vi "Module - Calibration.vi"(8 "Error In":errorcluster) -> (0 "Error Out":errorcluster)   [LabVIEW 2020]
uses:
  Control/State - Calibration.ctl
  Control/Cluster - Calibration Data.ctl
  Control/State - eFGV.ctl
  Control/Section Config RT.ctl
  <vilib>/Analysis/baseanly.llb/Mean (DBL).vi
  <vilib>/Analysis/NI_AALBase.lvlib
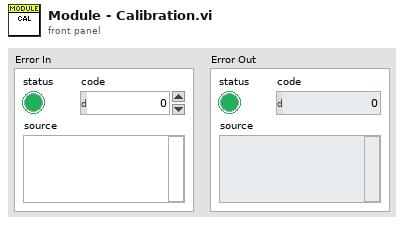
[diagram p1: front panel]
types:
  T1 = typedef "Cluster - Calibration Data.ctl" = cluster{"Slope":sgl, "Intercept":sgl, "Offset":sgl}
  T2 = cluster{"T_Out":i32, "AI Agg":waveform(dbl)[], "Calibration Data":T1[], "AI Calibrated":sgl[], "Event Ref":refnum<event-registration>, "Event - NS Connected":bool}
  T3 = typedef "State - Calibration.ctl" = enum16{"Init", "Register Event", "Read Calibration Config", "Idle", "Calibrate Sensor", "Close"}
  T4 = typedef "State - eFGV.ctl" = enum16{"Init", "Read", "Write", "Exit"}
  T5 = typedef "Section Config RT.ctl" = enum16{"Mod1/AI0", "Mod1/AI1", "Mod1/AI2", "Mod1/AI3", "Network Stream", "Acquisition Setting"}
  T6 = enum32{"invalid app kind", "Development System", "Run Time System", "Student Edition", "Embedded LabVIEW", "Evaluation", "Custom"}
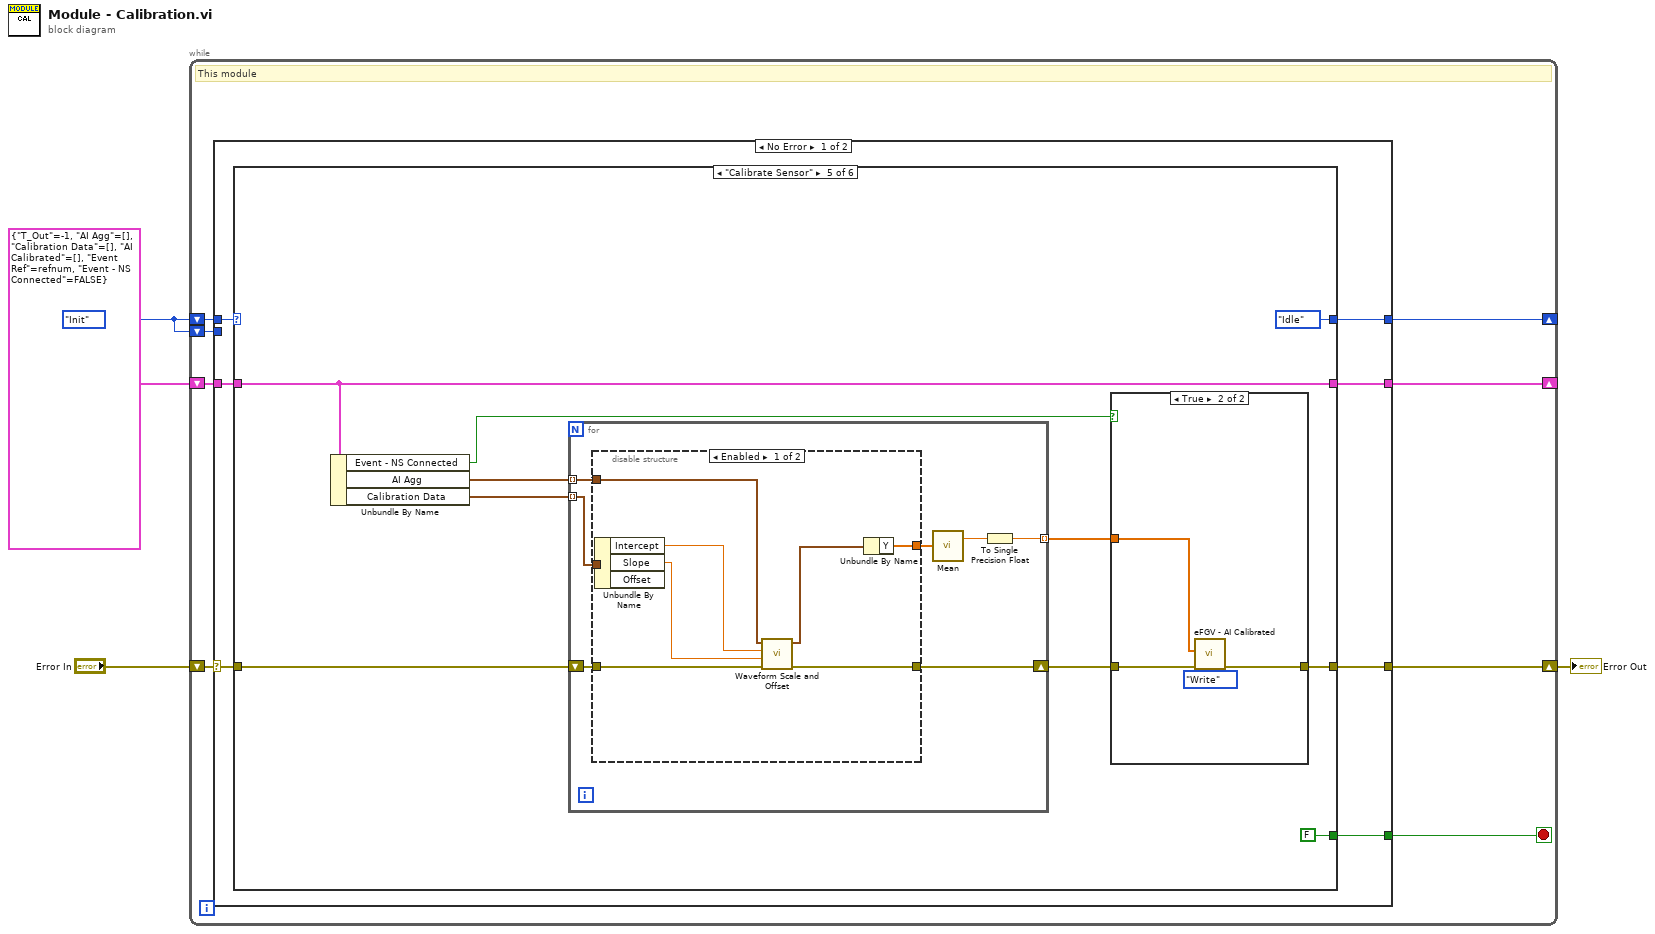
[diagram p0: block diagram]
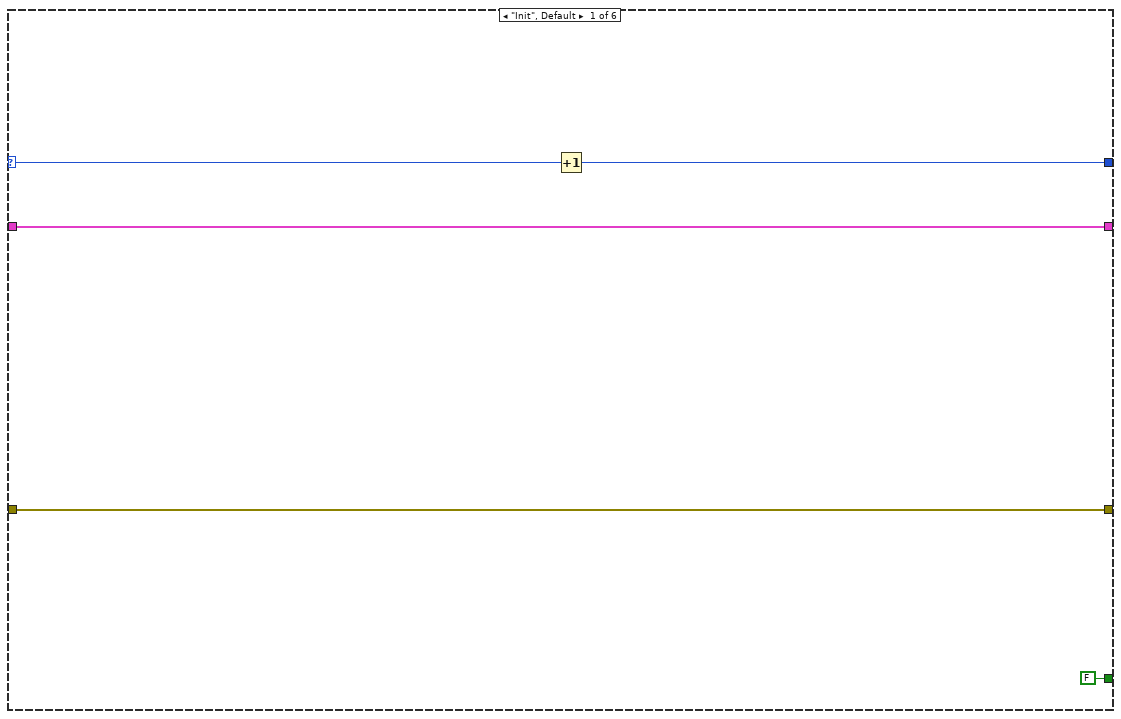
[diagram p2: hidden frame]
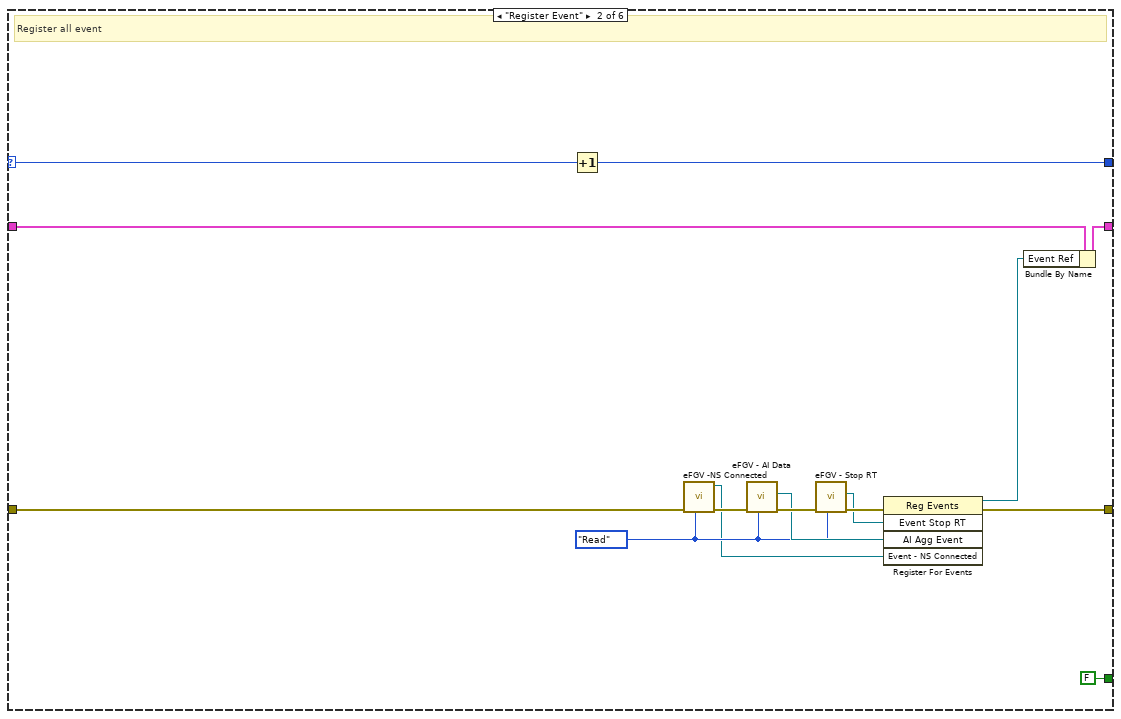
[diagram p3: hidden frame]
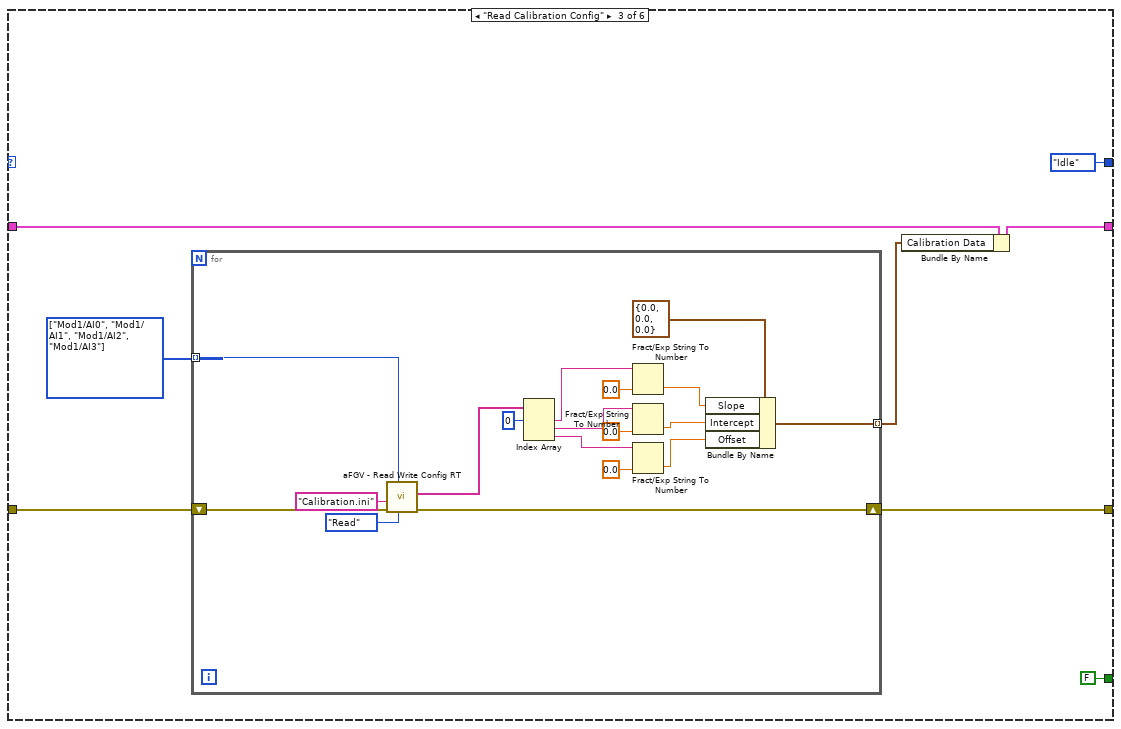
[diagram p4: hidden frame]
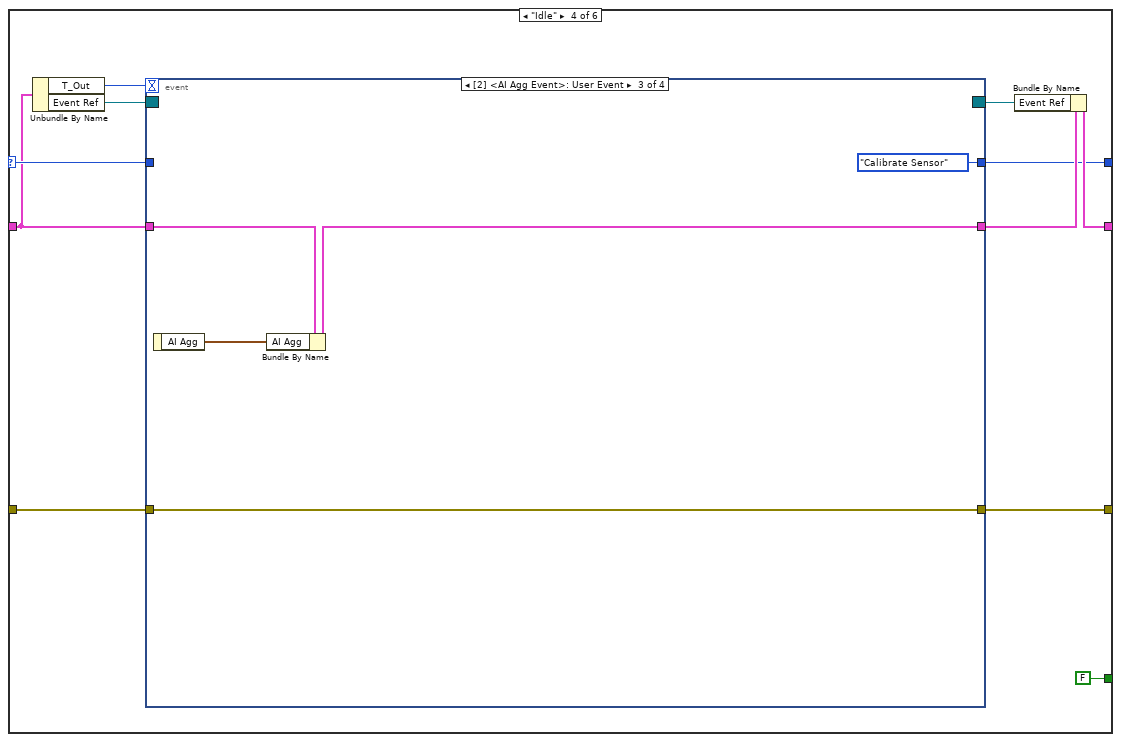
[diagram p5: hidden frame]
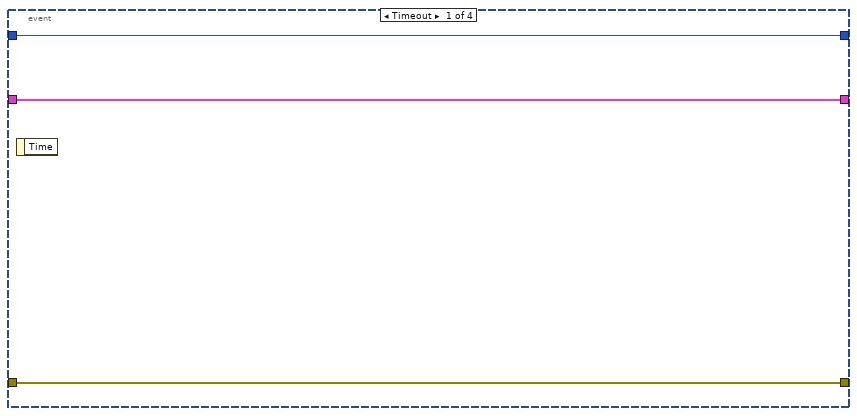
[diagram p6: hidden frame]
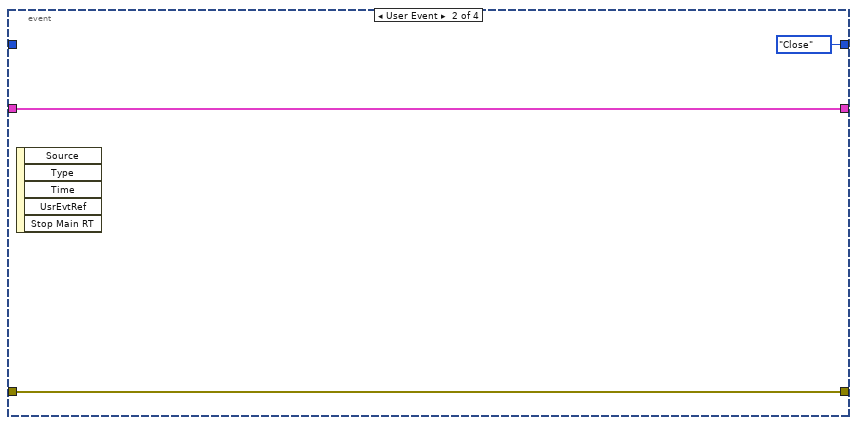
[diagram p7: hidden frame]
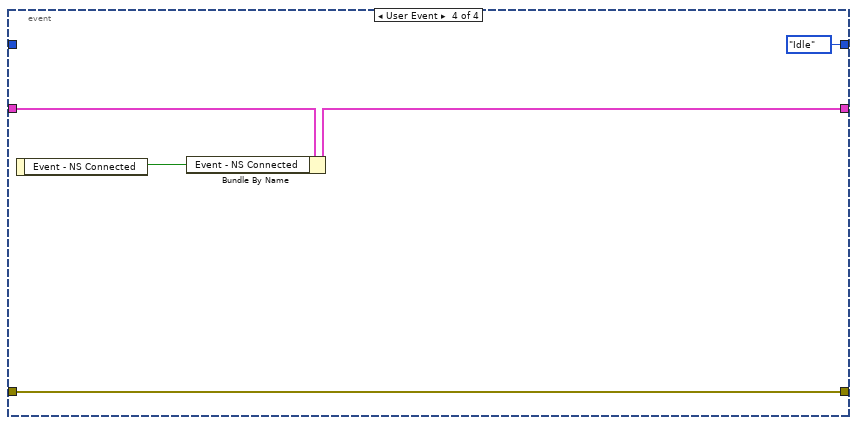
[diagram p8: hidden frame]
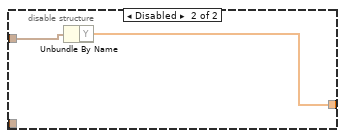
[diagram p10: hidden frame]
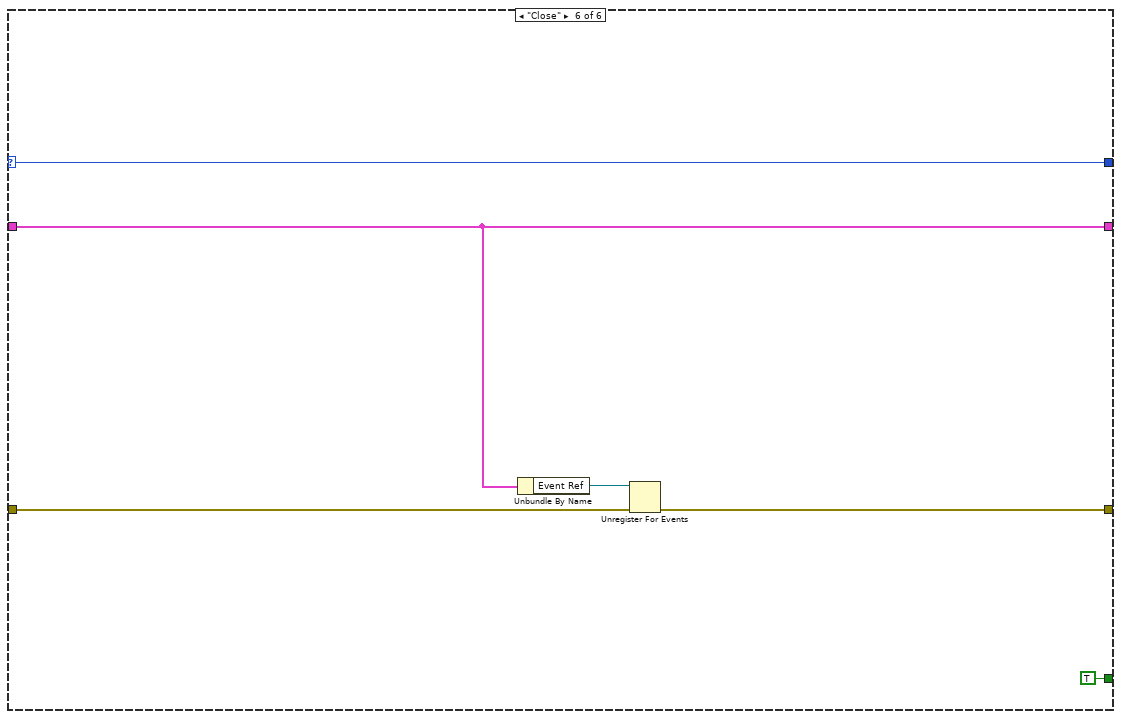
[diagram p11: hidden frame]
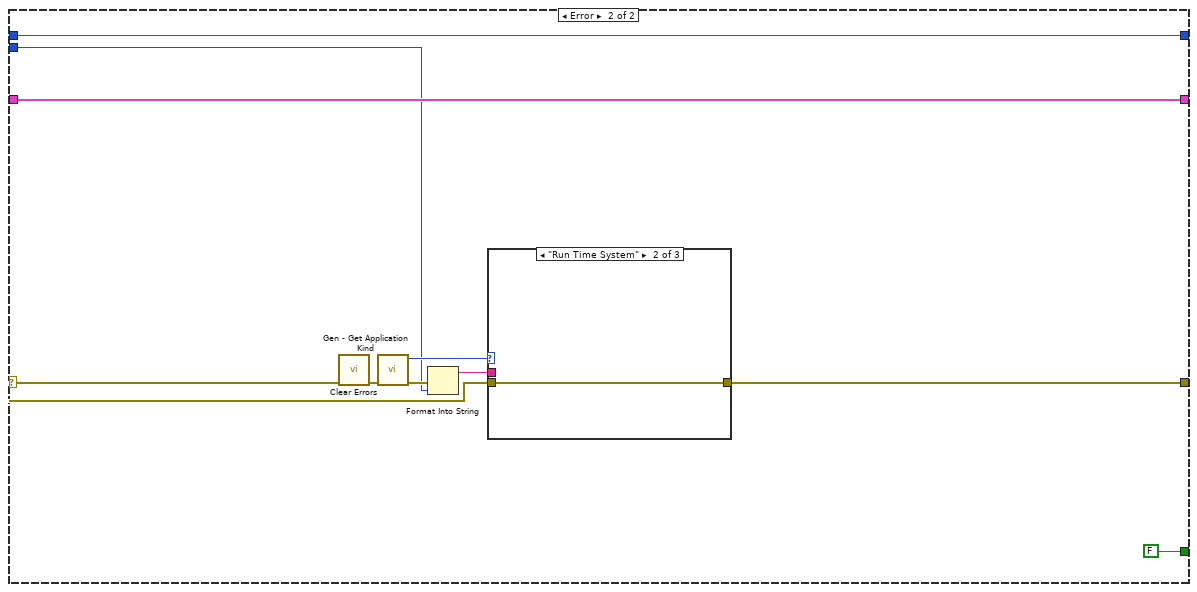
[diagram p12: hidden frame]
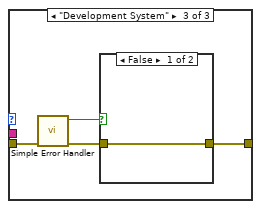
[diagram p14: hidden frame]
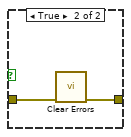
[diagram p15: hidden frame]
diagram:
  w1 = State_-_Calibration."Init"
  n1 = while {
    shift-right: [w8] -> _
    shift-left: w1 -> [w10]
    shift-right: [w11] -> w3
    shift-left: "Error In" -> [w12]
    shift-right: [w6] -> _
    shift-left: T2 {"T_Out"=-1, "AI Agg"=[], "Calibration Data"=[], "AI Calibrated"=[], "Event Ref"=refnum, "Event - NS Connected"=FALSE} -> [w7]
    shift-left: w1 -> [w5]
    stop <- w9 stop-if-true
    # "This module"
    n2 = case shown="No Error" w12 {
      selector: w12 -> [w19 w138]
      tunnel: w10 -> [w18 w135]
      tunnel: [w14 w139] -> w11
      tunnel: [w17 FALSE] -> w9
      tunnel: [w13 w135] -> w8
      tunnel: w7 -> [w16 w134]
      tunnel: [w15 w134] -> w6
      tunnel: w5 -> [_ w132]
      frame No Error {
        n3 = case shown="\"Calibrate Sensor\"" w18 {
          selector: w18 -> [w21 w31 _ w72 _ w128]
          tunnel: [w24 w39 w43 w76 w95 w129] -> w14
          tunnel: w19 -> [w24 w28 w44 w75 w99 w130]
          tunnel: [FALSE FALSE FALSE FALSE FALSE TRUE] -> w17
          tunnel: [w20 w30 State_-_Calibration."Idle" w66 State_-_Calibration."Idle" w128] -> w13
          tunnel: w16 -> [w23 w35 w47 w71 w100 w126]
          tunnel: [w23 w34 w41 w68 w100 w126] -> w15
          frame "Init", Default {
            n4 = Increment(x=w21) -> (x+1=w20:T3)
          }
          frame "Register Event" {
            w27 = State_-_eFGV."Read" ("State")
            # "Register all event"
            n5 = Increment(x=w31) -> (x+1=w30:T3)
            n6 = call "eFGV -NS Connected.vi"("States"=w27, "Error In"=w28) -> ("Error Out"=w29:errorcluster, "Event - NS Connected"=w26:refnum<user-event>)  [unwired: 8 in]
            n7 = call "eFGV - AI Data.vi"("States"=w27, "Error In"=w29) -> ("Error Out"=w33:errorcluster, "AI Agg Event"=w32:refnum<user-event>)  [unwired: 8 in]
            n8 = call "eFGV - Stop RT.vi"("State"=w27, "Error In"=w33) -> ("Error Out"=w38:errorcluster, "Event Stop RT"=w36:refnum<user-event>)  [unwired: 7 in, 1 out]
            n9 = register-events(error in=w38, w36, w32, w26) -> (reference out=w25:refnum<event-registration>, error out=w39:errorcluster)  [unwired: 1 in]
            n10 = Bundle By Name(cluster=w35, "Event Ref"=w25) -> (w34:T2)
          }
          frame "Read Calibration Config" {
            w42 = T5[] [enum."Mod1/AI0", enum."Mod1/AI1", enum."Mod1/AI2", enum."Mod1/AI3"] items=["Mod1/AI0", "Mod1/AI1", "Mod1/AI2", "Mod1/AI3", "Network Stream", "Acquisition Setting"] ("Array")
            n11 = for {
              shift-right: [w64] -> w43
              shift-left: w44 -> [w65]
              tunnel: w42 -> [w52] mode=indexing
              tunnel: [w48] -> w40 mode=indexing
              n12 = call "aFGV - Read Write Config RT.vi"("State"=enum16{"Read", "Write", "Delete"}."Read", "Section"=w52, "Error In"=w65, "File name"="Calibration.ini") -> ("Error Out"=w64:errorcluster, "Data out"=w62:string[])  [unwired: 5 in, 1 out]
              n13 = Index Array(array=w62, index #1=0 ("index")) -> (element #1=w51:string, element #2=w50:string, element #3=w49:string)  [unwired: 2 in]
              n14 = Fract/Exp String To Number(string=w51, default (0 dbl)=sgl 0.0 ("default (0 DBL)")) -> (number=w56:sgl)  [unwired: 2 in, 1 out]
              n15 = Fract/Exp String To Number(string=w50, default (0 dbl)=sgl 0.0 ("default (0 DBL)")) -> (number=w55:sgl)  [unwired: 2 in, 1 out]
              n16 = Fract/Exp String To Number(string=w49, default (0 dbl)=sgl 0.0 ("default (0 DBL)")) -> (number=w54:sgl)  [unwired: 2 in, 1 out]
              n17 = Bundle By Name(cluster=T1 {"Slope"=0.0, "Intercept"=0.0, "Offset"=0.0} ("Calibration Data"), "Slope"=w56, "Intercept"=w55, "Offset"=w54) -> (w48:T1)
            }
            n18 = Bundle By Name(cluster=w47, "Calibration Data"=w40) -> (w41:T2)
          }
          frame "Idle" {
            n19 = Unbundle By Name(w71) -> ("T_Out"=w70:i32, "Event Ref"=w69:refnum<event-registration>)
            n20 = event shown="[2] <AI Agg Event>: User Event" {
              selector: w69 -> [_ _ _ _]
              dyn-events: [_ _ _ _] -> w67
              timeout: w70 -> [_ _ _ _]
              tunnel: [w79 w82 w87 w92] -> w76
              tunnel: w75 -> [w79 w82 w87 w92]
              tunnel: [w77 State_-_Calibration."Close" State_-_Calibration."Calibrate Sensor" State_-_Calibration."Idle"] -> w66
              tunnel: [w78 w81 w84 w89] -> w73
              tunnel: w71 -> [w78 w81 w86 w91]
              tunnel: w72 -> [w77 _ _ _]
              event Timeout {
                n21 = event-data() -> ()  [unwired: 1 in, 1 out]
              }
              event User Event {
                n22 = event-data() -> ()  [unwired: 1 in, 5 out]
              }
              event User Event {
                n23 = event-data() -> ("AI Agg"=w83:waveform(dbl)[])  [unwired: 1 in]
                n24 = Bundle By Name(cluster=w86, "AI Agg"=w83) -> (w84:T2)
              }
              event User Event {
                n25 = event-data() -> ("Event - NS Connected"=w88:bool)  [unwired: 1 in]
                n26 = Bundle By Name(cluster=w91, "Event - NS Connected"=w88) -> (w89:T2)
              }
            }
            n27 = Bundle By Name(cluster=w73, "Event Ref"=w67) -> (w68:T2)
          }
          frame "Calibrate Sensor" {
            n28 = Unbundle By Name(w100) -> ("Event - NS Connected"=w93:bool, "AI Agg"=w98:waveform(dbl)[], "Calibration Data"=w97:T1[])
            n29 = for {
              shift-right: [w113] -> w96
              shift-left: w99 -> [w114]
              tunnel: w98 -> [w112] mode=indexing
              tunnel: w97 -> [w111] mode=indexing
              tunnel: [w108] -> w94 mode=indexing
              n30 = disable-structure shown="Enabled" {
                disable-tunnel: w114 -> [w122 _]
                disable-tunnel: [w121 _] -> w113
                disable-tunnel: w112 -> [w120 w124]
                disable-tunnel: w111 -> [w119 _]
                disable-tunnel: [w115 w123] -> w110
                frame Enabled {
                  n31 = Unbundle By Name(w119) -> ("Intercept"=w118:sgl, "Slope"=w117:sgl)  [unwired: 1 out]
                  n32 = call <vilib>:"Waveform Scale and Offset.vi"("error in (no error)"=w122, "scale"=w117, "offset"=w118, "waveform in"=w120) -> ("error out"=w121:errorcluster, "waveform out"=w116:waveform(dbl))  [unwired: 6 in]
                  n33 = Unbundle By Name(w116) -> ("Y"=w115:dbl[])
                }
                frame Disabled {
                  n34 = Unbundle By Name(w124) -> ("Y"=w123:dbl[])
                }
              }
              n35 = call-poly <vilib>:"Mean.vi"("X"=w110) -> ("mean"=w109:dbl)  [unwired: 1 out]
              n36 = To Single Precision Float(number=w109) -> (single precision float=w108:sgl)
            }
            n37 = case shown="True" w93 {
              tunnel: w96 -> [w103 w107]
              tunnel: [w103 w106] -> w95
              tunnel: w94 -> [_ w105]
              frame False {
              }
              frame True {
                n38 = call "eFGV - AI Calibrated.vi"("State"=State_-_eFGV."Write", "error in (no error)"=w107, "Event AI Calibrated"=w105) -> ("error out"=w106:errorcluster)  [unwired: 7 in, 1 out]
              }
            }
          }
          frame "Close" {
            n39 = Unbundle By Name(w126) -> ("Event Ref"=w125:refnum<event-registration>)
            n40 = Unregister For Events(event registration refnum=w125, error in=w130) -> (error out=w129:errorcluster)
          }
        }
      }
      frame Error {
        n41 = call <vilib>:"Clear Errors.vi"("error in (no error)"=w138) -> ("error out"=w140:errorcluster)  [unwired: 5 in, 1 out]
        n42 = call "Gen - Get Application Kind.vi"("Error In"=w140) -> ("Error Out"=w137:errorcluster, "Application:Kind"=w133:T6)  [unwired: 9 in]
        n43 = Format Into String(error in=w137, w132) -> (resulting string=w131:string)  [unwired: 2 in, 1 out]
        n44 = case shown="\"Run Time System\"" w133 {
          tunnel: [w141 w142 w146] -> w139
          tunnel: w138 -> [w141 w142 w144]
          tunnel: w131 -> [_ _ _]
          frame "invalid app kind", Default {
          }
          frame "Run Time System" {
          }
          frame "Development System" {
            n45 = call <vilib>:"Simple Error Handler.vi"("error in (no error)"=w144) -> ("error?"=w143:bool, "error out"=w145:errorcluster)  [unwired: 4 in, 3 out]
            n46 = case shown="False" w143 {
              tunnel: [w147 w149] -> w146
              tunnel: w145 -> [w147 w148]
              frame False {
              }
              frame True {
                n47 = call <vilib>:"Clear Errors.vi"("error in (no error)"=w148) -> ("error out"=w149:errorcluster)  [unwired: 5 in, 1 out]
              }
            }
          }
        }
      }
    }
  }
  "Error Out" <- w3
